vi "ConfigAcquisition.vi"(8 "error in (no error)":errorcluster, 11 "Infiniium in":refnum<class "Infiniium.lvclass">) -> (0 "error out":errorcluster, 3 "Infiniium out":refnum<class "Infiniium.lvclass">)   [LabVIEW 2018]
uses:
  <vilib>/Utility/error.llb/Error Cluster From Error Code.vi
  <vilib>/ErrorRing/Error Ring.xnode
  <instrlib>/Agilent 90000 Series/Agilent 90000 Series.lvlib
  Infiniium.lvclass
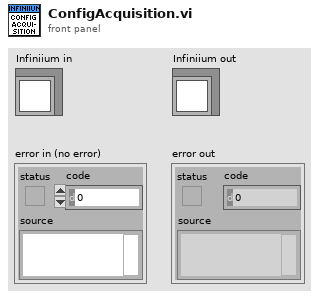
[diagram p1: front panel]
types:
  T1 = typedef "ScopePlugins.lvlib/Acquisition.ctl" = cluster{"StartTime":dbl, "Type":enum16{"Normal", "PeakDetect", "HighRes", "Envelope", "Average"}, "NumPointsMin":i32, "RecordLength":i32, "SampleRate":dbl, "TimePerRecord":dbl, "SamplingMode ":enum16{"Real Time", "Equivalent Time", "Segment", "Real Time Peak Detect", "Real Time High Resolution", "Peak Detect Segment", "High Resolution Segment"}, "Interpolation":enum16{"No Interpolation", "sin(x)/x", "linear", "1 Point sin(x)/x", "2 Point sin(x)/x", "4 Point sin(x)/x", "8 Point sin(x)/x", "16 Point sin(x)/x"}, "NumAverages":i32, "Resolution":enum16{"Auto", "Bits 9", "Bits 10", "Bits 11", "Bits 12"}, "EnableAveraging":bool, "Continuous":bool}
  T2 = enum16{"Real Time", "Equivalent Time", "Segment", "Real Time Peak Detect", "Real Time High Resolution", "Peak Detect Segment", "High Resolution Segment"}
  T3 = enum16{"No Interpolation", "sin(x)/x", "linear", "1 Point sin(x)/x", "2 Point sin(x)/x", "4 Point sin(x)/x", "8 Point sin(x)/x", "16 Point sin(x)/x"}
  T4 = enum16{"Auto", "Bits 9", "Bits 10", "Bits 11", "Bits 12"}
  T5 = enum16{"Normal", "PeakDetect", "HighRes", "Envelope", "Average"}
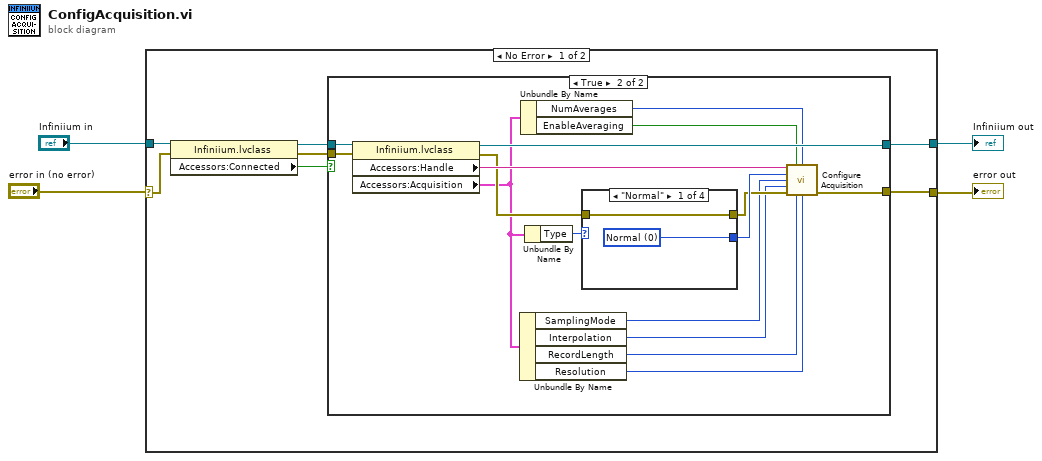
[diagram p0: block diagram]
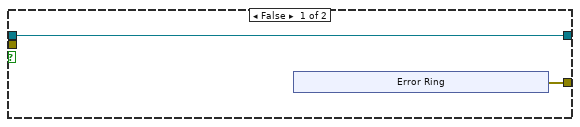
[diagram p2: hidden frame]
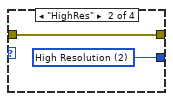
[diagram p3: hidden frame]
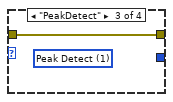
[diagram p4: hidden frame]
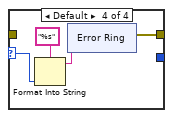
[diagram p5: hidden frame]
diagram:
  n1 = case shown="No Error" "error in (no error)" {
    selector: "error in (no error)" -> [w10 w52]
    tunnel: [w6 w52] -> w3
    tunnel: [w5 w51] -> w1
    tunnel: "Infiniium in" -> [w11 w51]
    frame No Error {
      n2 = property class="Infiniium.lvclass"(reference=w11, error in=w10) -> (reference out=w9:refnum<class "Infiniium.lvclass">, error out=w8:errorcluster, "Accessors:Connected"=w7:bool)
      n3 = case shown="True" w7 {
        tunnel: w9 -> [w12 w33]
        tunnel: w8 -> [_ w34]
        tunnel: [w13 w24] -> w6
        tunnel: [w12 w31] -> w5
        frame False {
          n4 = xnode "Error Ring"() -> ("error out"=w13:errorcluster)
        }
        frame True {
          n5 = property class="Infiniium.lvclass"(reference=w33, error in=w34) -> (reference out=w31:refnum<class "Infiniium.lvclass">, error out=w27:errorcluster, "Accessors:Handle"=w32:string, "Accessors:Acquisition"=w21:T1)
          n6 = Unbundle By Name(w21) -> ("SamplingMode"=w23:T2, "Interpolation"=w22:T3, "RecordLength"=w20:i32, "Resolution"=w19:T4)
          n7 = Unbundle By Name(w21) -> ("NumAverages"=w30:i32, "EnableAveraging"=w29:bool)
          n8 = Unbundle By Name(w21) -> ("Type"=w28:T5)
          n9 = case shown="\"Normal\"" w28 {
            selector: w28 -> [_ _ _ w41]
            tunnel: [w36 w38 _ _] -> w26
            tunnel: w27 -> [w35 w37 w39 _]
            tunnel: [w35 w37 w39 w43] -> w25
            frame "Normal" {
              w36 = 0 items=["Normal", "Peak Detect", "High Resolution"] ("Acquisition Type (0: Normal)")
            }
            frame "HighRes" {
              w38 = 2 items=["Normal", "Peak Detect", "High Resolution"] ("Acquisition Type (0: Normal)")
            }
            frame "PeakDetect" {
              (unwired) 1 items=["Normal", "Peak Detect", "High Resolution"] ("Acquisition Type (0: Normal)")
            }
            frame Default {
              n10 = Format Into String(format string="%s", w41) -> (resulting string=w42:string)  [unwired: 2 in, 1 out]
              n11 = xnode "Error Ring"("parameter 0"=w42) -> ("error out"=w43:errorcluster)
            }
          }
          n12 = call <instrlib>:"Configure Acquisition.vi"("VISA resource name"=w32, "Enable Analog Averaging (Disable)"=w29, "Number Of Averages (8)"=w30, "Acquisition Type (0: Normal)"=w26, "Sampling Mode  (0: Real Time)"=w23, "Interpolation (0:No Interpolation)"=w22, "error in (no error)"=w25, "Segment Count (256)"=w20, "Resolution (0:Auto)"=w19) -> ("error out"=w24:errorcluster)  [unwired: 5 in, 1 out]
        }
      }
    }
    frame Error {
    }
  }
  "error out" <- w3
  "Infiniium out" <- w1
